vi "File dir to Image dir.vi"(0 "Documentation Folder":path, 1 "Image Folder":path, 4 "File":path caption="File Directory") -> (6 "Folder":path, 7 "File":string, 9 "Type":string)   [LabVIEW 2017, in "DocTools.lvlib"]
uses:
  DocTools.lvlib
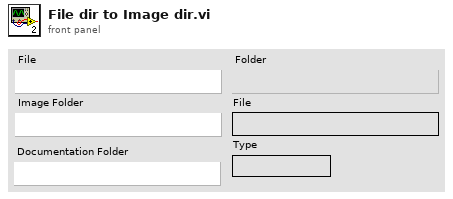
[diagram p1: front panel]
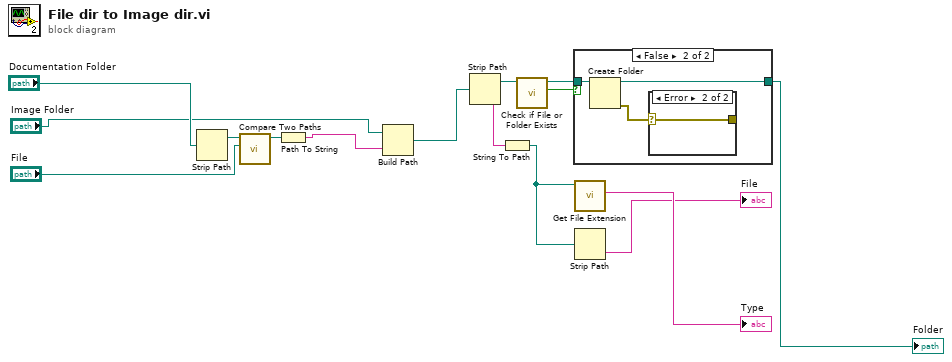
[diagram p0: block diagram]
diagram:
  n1 = Strip Path(path="Documentation Folder") -> (stripped path=w15:path)  [unwired: 1 out]
  n2 = call <vilib>:"Compare Two Paths.vi"("Path 2"="File", "Path 1"=w15) -> ("Relative Path from 1 to 2"=w14:path)  [unwired: 6 in, 3 out]
  n3 = Path To String(path=w14) -> (string=w13:string)
  n4 = Build Path(base path="Image Folder", name or relative path=w13) -> (appended path=w11:path)
  n5 = Strip Path(path=w11) -> (stripped path=w10:path, name=w6:string)
  n6 = String To Path(string=w6) -> (path=w2:path)
  n7 = call <vilib>:"Check if File or Folder Exists.vi"("path"=w10) -> ("file or folder exists?"=w9:bool, "dup path"=w8:path)  [unwired: 8 in, 1 out]
  n8 = case shown="False" w9 {
    tunnel: w8 -> [w16 w19]
    tunnel: [w16 w18] -> w7
    frame True {
    }
    frame False {
      n9 = Create Folder(path (use dialog)=w19) -> (created path=w18:path, error out=w17:errorcluster)  [unwired: 2 in, 1 out]
      n10 = case shown="Error" w17 {
        selector: w17 -> [w20 w21]
        tunnel: [w20 w21] -> _
        frame No Error {
        }
        frame Error {
        }
      }
    }
  }
  "Folder" <- w7
  n11 = call <vilib>:"Get File Extension.vi"("file"=w2) -> ("lowercase file extension"=→"Type":string)  [unwired: 6 in, 4 out]
  n12 = Strip Path(path=w2) -> (name=→"File":string)  [unwired: 1 out]
